vi "GetDescription.vi"(9 "Error in":errorcluster) -> (1 "Description":string)   [LabVIEW 2017, in "GPError.lvlib"]
doc: "Returns <B>Description</B> derived from <B>Error in</B>. For appended errors the description from the primary error/warning is returned only.\n\nThis VI builds the description either from the description part of the Source field of <B>Error in</B>, by getting a built-in description, or by building a custom or compound description if given.\n\nThis VI is inlined.\n\nSteen Schmidt\nGPower\n17/11 2012"
uses:
  GPError.lvlib
panel:
  # "Copyright © 2013\nSteen Schmidt, GPower\nSee enclosed license file for terms and conditions"
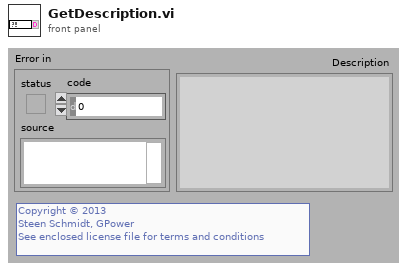
[diagram p1: front panel]
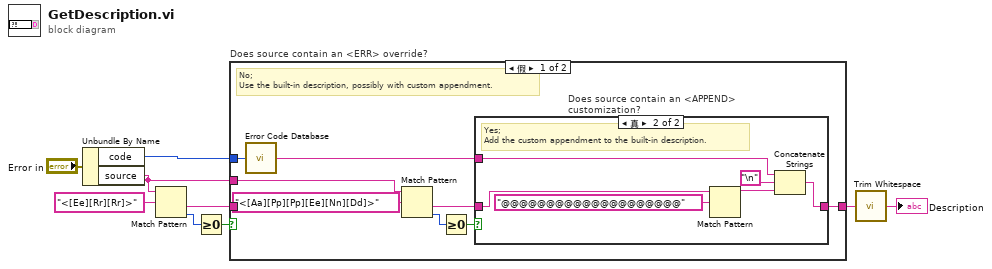
[diagram p0: block diagram]
diagram:
  n1 = Unbundle By Name("Error in") -> ("code"=w5:i32, "source"=w4:string)
  n2 = Match Pattern(string=w4, regular expression="<[Ee][Rr][Rr]>") -> (after substring=w6:string, offset past match=w8:i32)  [unwired: 1 in, 2 out]
  n3 = Greater Or Equal To 0?(x=w8) -> (x >= 0?=w7:bool)
  n4 = case "Does source contain an <ERR> override?" shown="假" w7 {
    tunnel: w6 -> [_ w25]
    tunnel: [w10 w25] -> w3
    tunnel: w5 -> [w17 _]
    tunnel: w4 -> [w15 _]
    frame False {
      # "No;\nUse the built-in description, possibly with custom appendment."
      n5 = call <vilib>:"Error Code Database.vi"("Error Code"=w17) -> ("Error Text"=w11:string)
      n6 = Match Pattern(string=w15, regular expression="<[Aa][Pp][Pp][Ee][Nn][Dd]>") -> (after substring=w12:string, offset past match=w14:i32)  [unwired: 1 in, 2 out]
      n7 = Greater Or Equal To 0?(x=w14) -> (x >= 0?=w13:bool)
      n8 = case "Does source contain an <APPEND> customization?" shown="真" w13 {
        tunnel: w12 -> [_ w24]
        tunnel: w11 -> [w18 w20]
        tunnel: [w18 w21] -> w10
        frame False {
          # "No;\nJust use the built-in description."
        }
        frame True {
          # "Yes;\nAdd the custom appendment to the built-in description."
          n9 = Match Pattern(string=w24, regular expression="@@@@@@@@@@@@@@@@@@@@") -> (before substring=w22:string)  [unwired: 1 in, 3 out]
          n10 = Concatenate Strings(w20, "\n", w22) -> (w21:string)
        }
      }
    }
    frame True {
      # "Yes;\nThe <ERR> override is the description."
    }
  }
  n11 = call <vilib>:"Trim Whitespace.vi"("string"=w3) -> ("trimmed string"=→"Description":string)  [unwired: 1 in]
